vi "Arm Controls.vi"(11 "Robot Commands":T1) -> ()   [LabVIEW 2014]
uses:
  SubSystems/Robot Commands.ctl
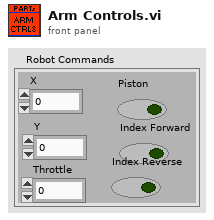
[diagram p1: front panel]
types:
  T1 = typedef "Robot Commands.ctl" = cluster{"X":dbl, "Y ":dbl, "Throttle":dbl, "Piston":bool, "Index Forward":bool, "Index Reverse ":bool}
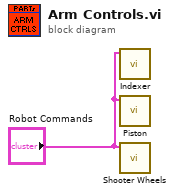
[diagram p0: block diagram]
diagram:
  n1 = call "Indexer.vi"("Robot Commands"="Robot Commands") -> ()  [unwired: 11 in]
  n2 = call "Piston.vi"("Robot Commands"="Robot Commands") -> ()  [unwired: 11 in]
  n3 = call "Shooter Wheels.vi"("Robot Commands"="Robot Commands") -> ()  [unwired: 11 in]
